vi "AI Notifier.vi"(11 "Action":enum16{"Get", "Set"}(ring)) -> (3 "Trigger?":bool)   [LabVIEW 2021]
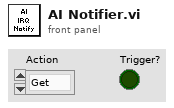
[diagram p1: front panel]
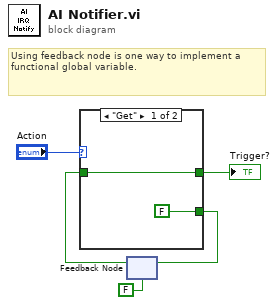
[diagram p0: block diagram]
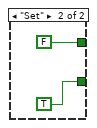
[diagram p2: hidden frame]
diagram:
  # "Using feedback node is one way to implement a functional global variable."
  n1 = feedback #1(FALSE ("Boolean")) -> (w1:bool)
  n2 = case shown="\"Get\"" "Action" {
    tunnel: [w7 FALSE ("Boolean")] -> w5
    tunnel: [FALSE TRUE] -> w2
    tunnel: w1 -> [w7 _]
    frame "Get" {
    }
    frame "Set" {
    }
  }
  "Trigger?" <- w5
  n3 = feedback-in #1(w2) -> ()
